vi "Robot Global Data.vi"() -> ()   [LabVIEW 2019]
doc: "This global VI can contain as many global variables as you need. To create a global variable, place a control on the panel, give it a good name. To read or write to it from a VI, drag the icon to the diagram of that VI. You can also drag from the project. Click on the node to change which global you access. You shouldn't have multiple locations writing to a global or it will cause a race-condition."
uses:
  <vilib>/Rock Robotics/WPI/Camera/WPI_CameraImageSize.ctl
  <vilib>/Rock Robotics/WPI/DriverStation/WPI_DriverStationRobotMode2.ctl
  Shooter/Implementation/Shooter Operations.ctl
panel:
  in  "LEDS":bool
  in  "First path":bool
  in  "Shot Position":dbl
  in  "Reverse Intake?":bool
  in  "Hold Intake down?":bool
  in  "POVs?":bool
  in  "Shooter Operation":T1
  in  "Intake up for __ secs?":bool
  in  "Transfer Full?":bool
  in  "Reset Transfer":bool
  in  "Feeder Station Vision":bool
  in  "Auto":path[](array[path])
  in  "Reset?":bool
  in  "Shoot":bool
  in  "Turret AA":dbl
  in  "AD Drivebase":cluster{"Right":string, "Left":string}[](array[cluster])
  in  "AD Disabled":string[](array[string])
  in  "Ball AA":dbl
  in  "Robot Mode":T2
  in  "image size":T3=enum."320x240"
  in  "Ball Vision":bool
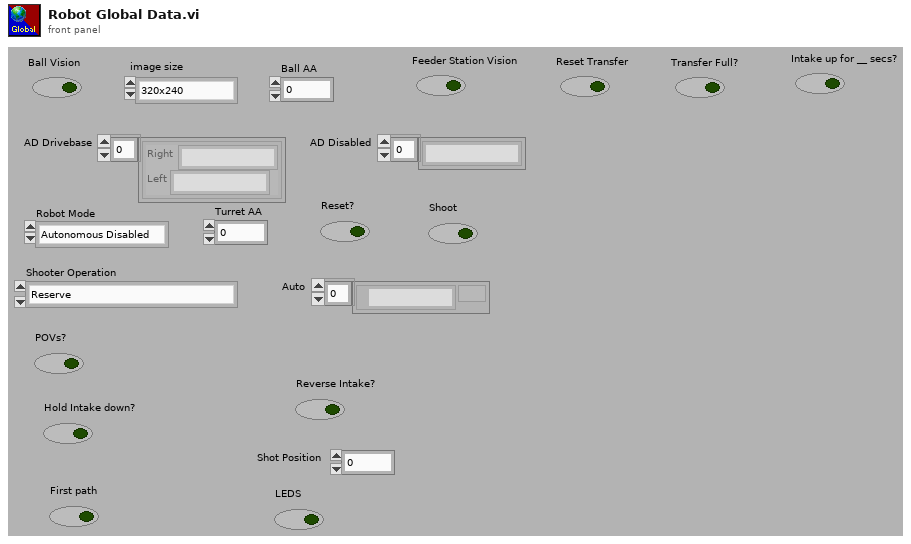
[diagram p1: front panel]
types:
  T1 = typedef "Shooter Operations.ctl" = enum16{"Reserve", "Read Current", "Immediate"}
  T2 = typedef "WPI_DriverStationRobotMode2.ctl" = enum16{"Autonomous Disabled", "Autonomous Enabled", "Teleop Disabled", "Teleop Enabled", "Disconnected", "Finish", "Test Disabled", "Test Enabled", "Emergency Stopped"}
  T3 = typedef "WPI_CameraImageSize.ctl" = enum16{"640x480", "320x240", "160x120", "Custom"}
diagram:
